vi "Configure Dialog.vi"(8 "error in (no error)":errorcluster, 11 "Clear Arbitrary Memory [SEQ] Msg.lvclass":refnum<class "Clear Arbitrary Memory [SEQ] Msg.lvclass">) -> (0 "error out":errorcluster, 2 "Ok?":bool, 3 "Clear Arbitrary Memory [SEQ] Msg.lvclass":refnum<class "Clear Arbitrary Memory [SEQ] Msg.lvclass">)   [LabVIEW 2015, in "CS++Fgen.lvlib" / "Clear Arbitrary Memory [SEQ] Msg.lvclass"]
uses:
  Clear Arbitrary Memory [SEQ] Msg.lvclass
  Clear Arbitrary Memory [SEQ] Msg.lvclass/Clear Arbitrary Memory [SEQ] Msg.ctl
panel:
  in  "Cancel Button":bool
  in  "OK Button":bool
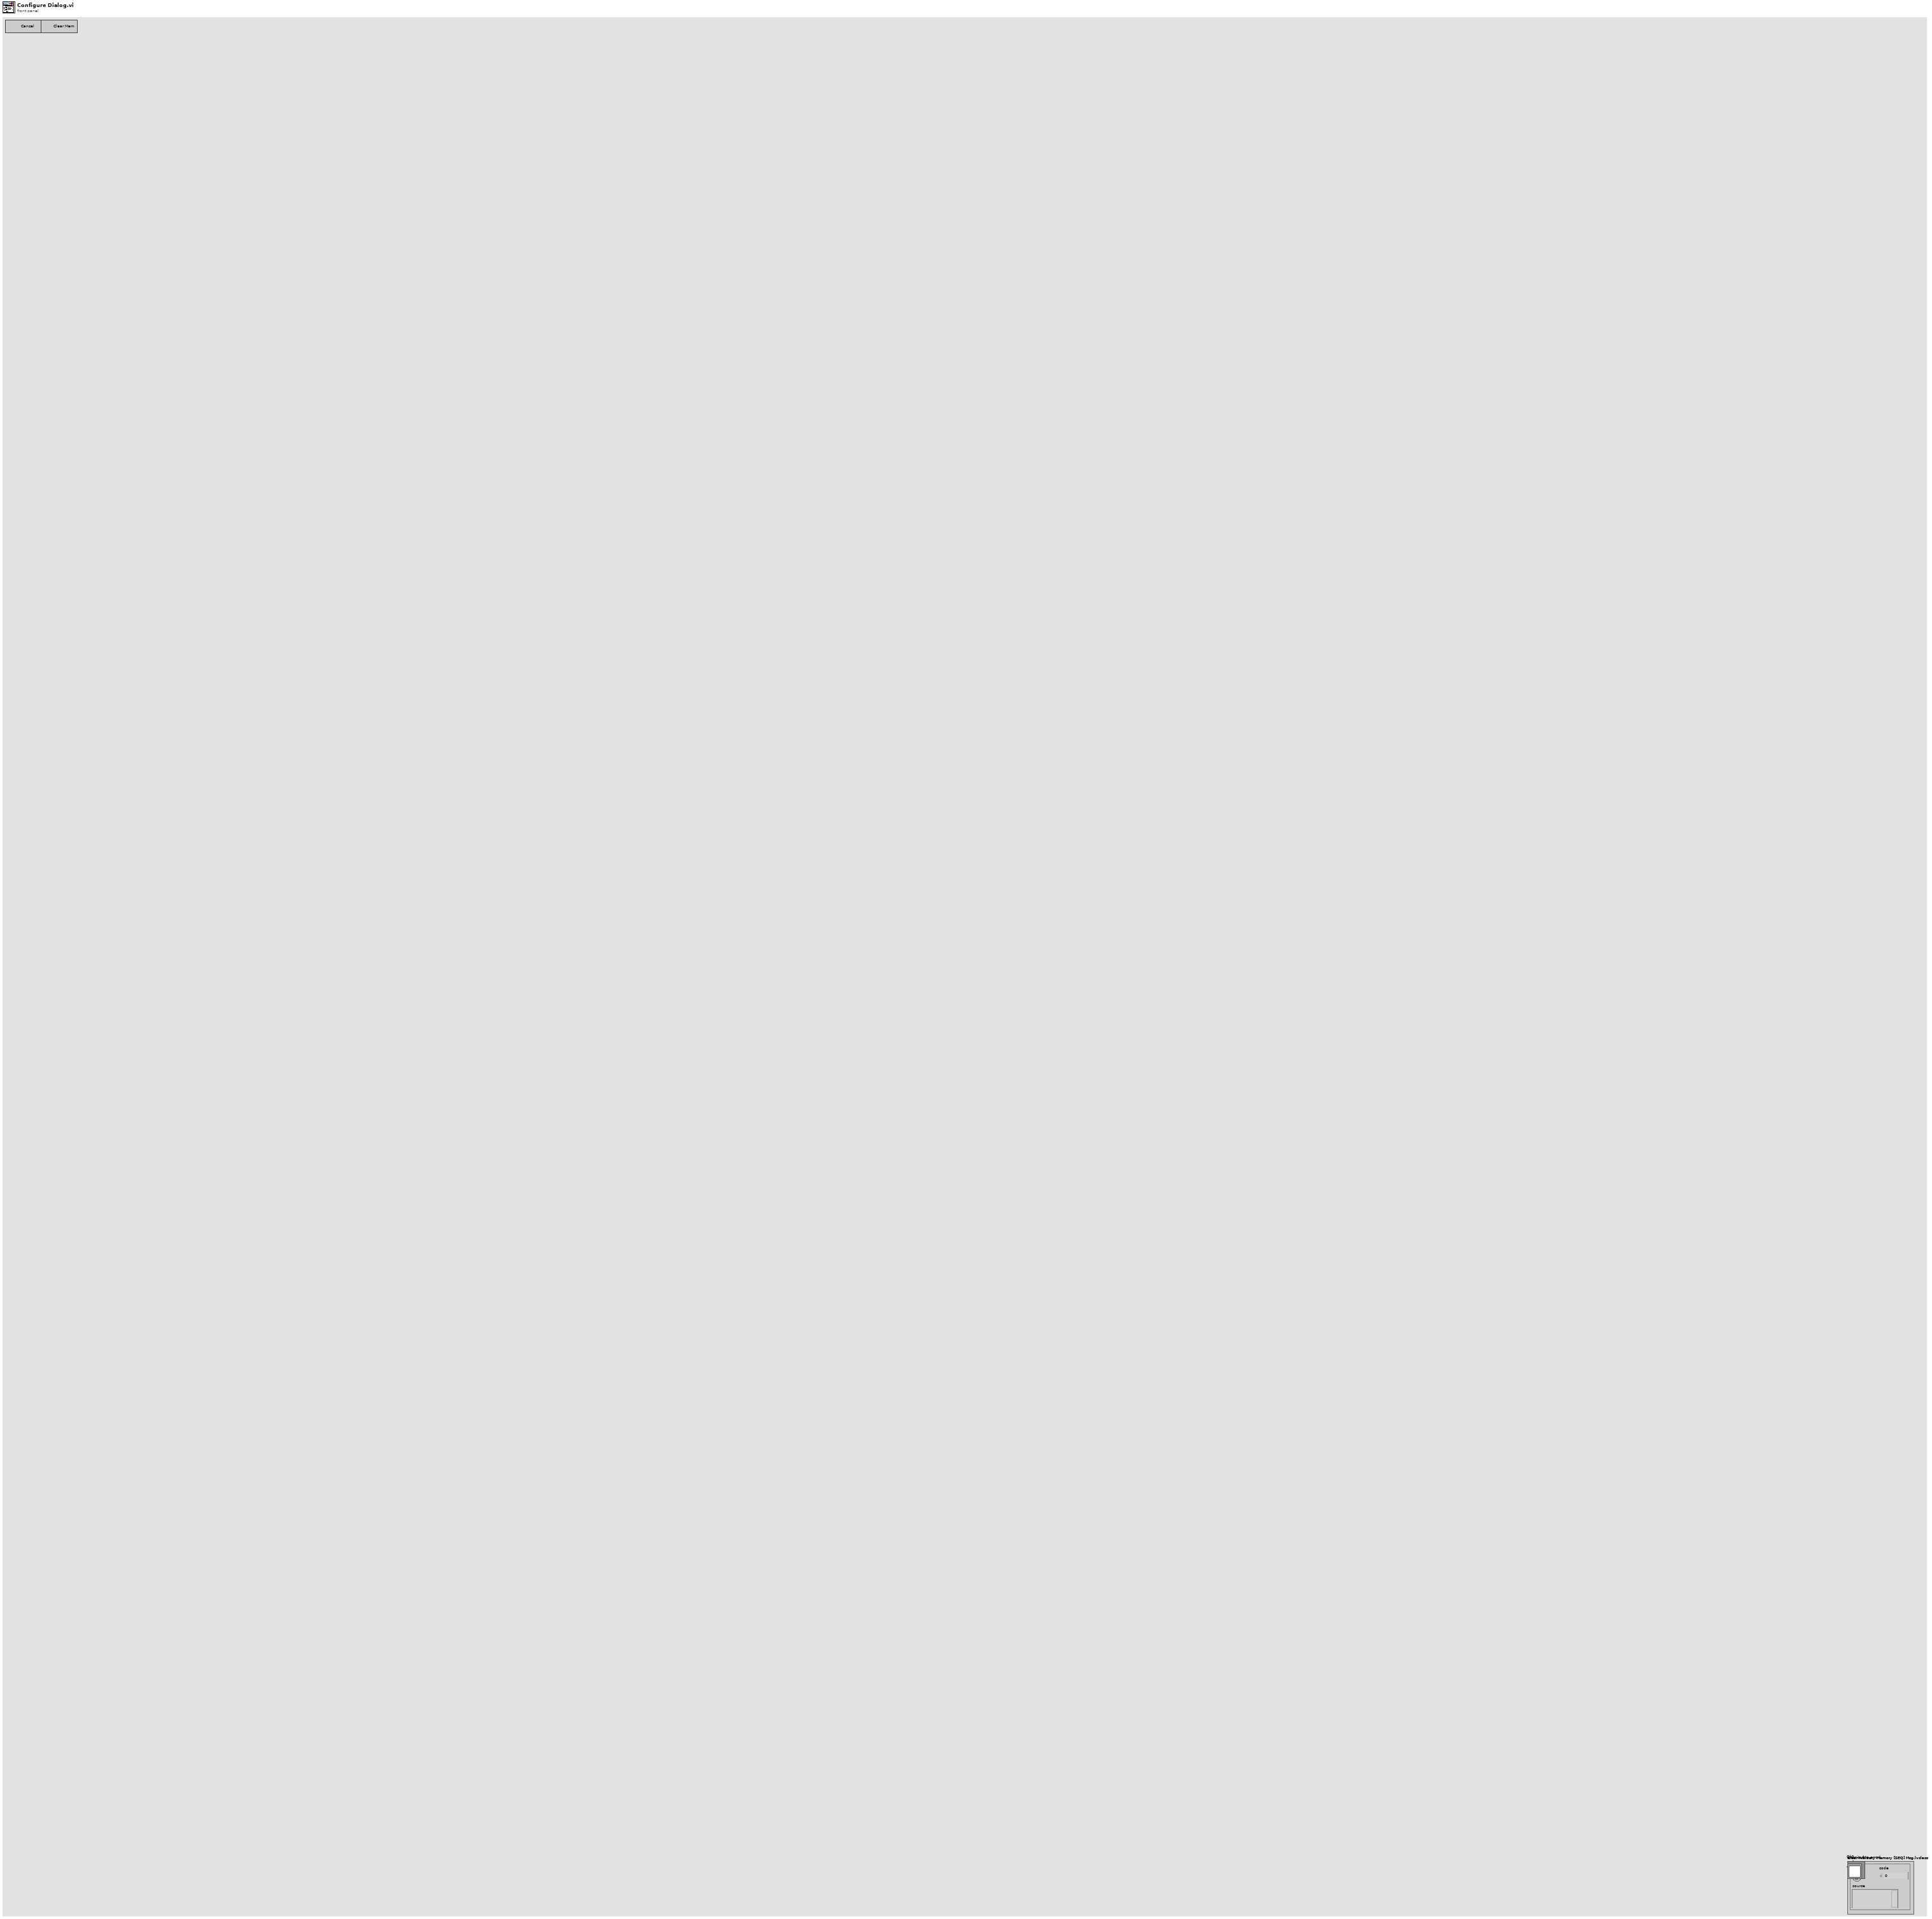
[diagram p1: front panel]
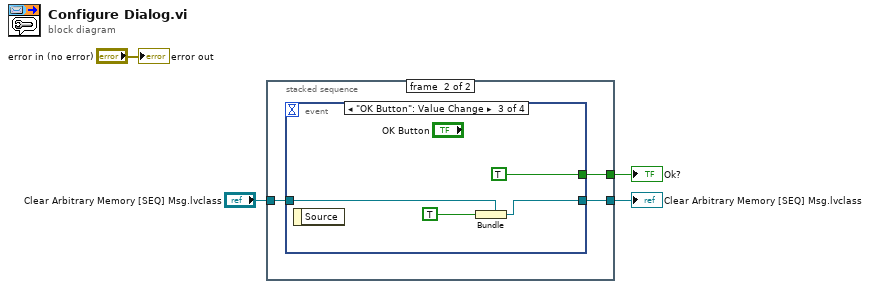
[diagram p0: block diagram]
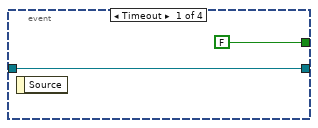
[diagram p3: hidden frame]
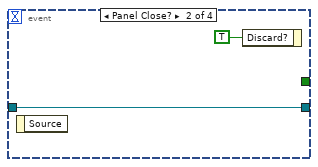
[diagram p4: hidden frame]
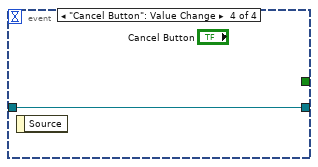
[diagram p5: hidden frame]
diagram:
  n1 = stacked-sequence {
    tunnel: [_ w7] -> w3
    tunnel: [_ w6] -> w2
    tunnel: "Clear Arbitrary Memory [SEQ] Msg.lvclass" -> [_ w5]
    frame #0 {
    }
    frame #1 {
      n2 = event shown="[2] \"OK Button\": Value Change" {
        selector: _ -> [_ _ _ _]
        dyn-events: _ -> [_ _ _ _]
        timeout: _ -> [_ _ _ _]
        tunnel: [w8 w10 w13 w16] -> w6
        tunnel: w5 -> [w8 w10 w15 w16]
        tunnel: [FALSE _ TRUE _] -> w7
        event Timeout {
          n3 = event-data() -> ()  [unwired: 1 in, 1 out]
        }
        event Panel Close? {
          n4 = event-data() -> ()  [unwired: 1 in, 1 out]
          n5 = event-data ("Event Filter Node")("Discard?"=TRUE) -> ()  [unwired: 1 in, 1 out]
        }
        event "OK Button": Value Change {
          n6 = event-data() -> ()  [unwired: 1 in, 1 out]
          n7 = Bundle ("Main-Bundler")(cluster=w15, TRUE ("Execute?")) -> (w13:refnum<class "Clear Arbitrary Memory [SEQ] Msg.lvclass">)
        }
        event "Cancel Button": Value Change {
          n8 = event-data() -> ()  [unwired: 1 in, 1 out]
        }
      }
    }
  }
  "Ok?" <- w3
  "Clear Arbitrary Memory [SEQ] Msg.lvclass" <- w2
  "error out" <- "error in (no error)"
